vi "helper - UTM line to Square.vi"(2 "Endpoint 2, UTM":T1 {"North" format="%#_10f"; "East" format="%#_8f"}, 3 "Endpoint 1, UTM":T1 {"North" format="%#_10f"; "East" format="%#_8f"}) -> (0 "Endpoint 4, UTM":T1 {"North" format="%#_10f"; "East" format="%#_8f"}, 1 "Endpoint 3, UTM":T1 {"North" format="%#_10f"; "East" format="%#_8f"})   [LabVIEW 2011]
doc: "takes in an ROI such as that produced by the line tool, along with an image descriptor, and outputs the UTM locations of the line's endpoints."
uses:
  2-Think/2 Typedefs/UTM Location.ctl
  2-Think/2 Typedefs/heading.ctl
panel:
  in  "check with graph":bool
  out "XY Graph":cluster{dbl[], dbl[]}(graph)
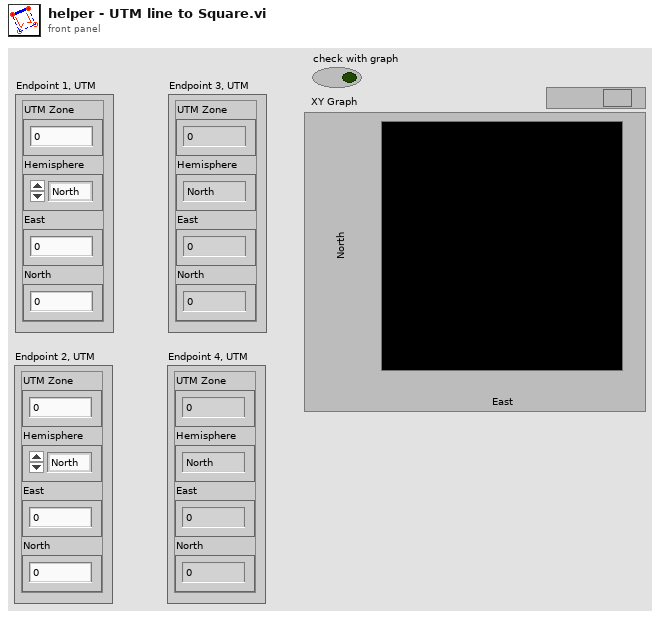
[diagram p1: front panel]
types:
  T1 = typedef "UTM Location.ctl" = cluster{"UTM Zone":dbl, "Hemisphere":enum16{"North", "South"}, "East":dbl, "North":dbl}
  T2 = typedef "heading.ctl" = dbl
  T3 = typedef "Velocity.ctl" = cluster{"East":dbl, "North":dbl}
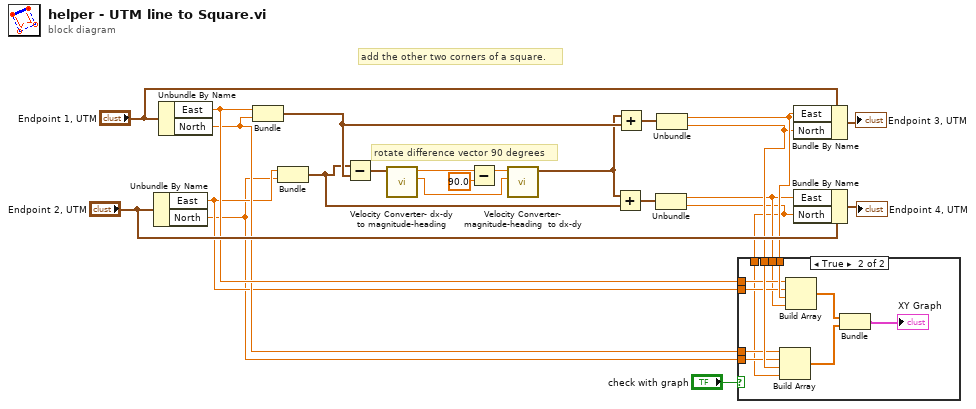
[diagram p0: block diagram]
diagram:
  # "rotate difference vector 90 degrees"
  # "add the other two corners of a square."
  n1 = Unbundle By Name("Endpoint 2, UTM") -> ("East"=w10:dbl, "North"=w9:dbl)
  n2 = Unbundle By Name("Endpoint 1, UTM") -> ("East"=w12:dbl, "North"=w11:dbl)
  n3 = Bundle("East"=w12, "North"=w11) -> (w7:cluster{"East":dbl, "North":dbl})  [unwired: 1 in]
  n4 = Bundle("East"=w10, "North"=w9) -> (w2:cluster{"East":dbl, "North":dbl})  [unwired: 1 in]
  n5 = Subtract ("Difference\nVector")(x=w2, y=w7) -> (x-y=w8:cluster{"East":dbl, "North":dbl})
  n6 = call "Velocity Converter- dx-dy to magnitude-heading.vi"("Vector In"=w8) -> ("Magnitude Out"=w16:dbl, "Heading Out"=w18:T2)  [unwired: 9 in]
  n7 = Subtract(x=w18, y=T2 90.0 ("x")) -> (x-y=w17:T2)
  n8 = call "Velocity Converter- magnitude-heading  to dx-dy.vi"("Magnitude"=w16, "Heading"=w17) -> ("Vector Out"=w3:T3)  [unwired: 9 in]
  n9 = Add(x=w3, y=w2) -> (x+y=w6:T3)
  n10 = Add(x=w3, y=w7) -> (x+y=w15:T3)
  n11 = Unbundle(w6) -> ("East"=w5:dbl, "North"=w4:dbl)
  n12 = Unbundle(w15) -> ("East"=w14:dbl, "North"=w13:dbl)
  n13 = case shown="True" "check with graph" {
    tunnel: w14 -> [_ w31]
    tunnel: w13 -> [_ w30]
    tunnel: w12 -> [_ w29]
    tunnel: w11 -> [_ w28]
    tunnel: w10 -> [_ w27]
    tunnel: w9 -> [_ w26]
    tunnel: w5 -> [_ w25]
    tunnel: w4 -> [_ w24]
    frame False {
    }
    frame True {
      n14 = Build Array(w28, w26, w30, w24) -> (w33:dbl[])
      n15 = Build Array(w29, w27, w31, w25) -> (w34:dbl[])
      n16 = Bundle(w34, w33) -> (→"XY Graph":cluster{dbl[], dbl[]})  [unwired: 1 in]
    }
  }
  n17 = Bundle By Name(cluster="Endpoint 1, UTM", "East"=w14, "North"=w13) -> (→"Endpoint 3, UTM":T1)
  n18 = Bundle By Name(cluster="Endpoint 2, UTM", "East"=w5, "North"=w4) -> (→"Endpoint 4, UTM":T1)
